vi "4CHDAQ - Check Text File Name.vi"(11 "path":path) -> (3 "Error Type":i32)   [LabVIEW 2015]
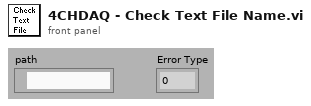
[diagram p1: front panel]
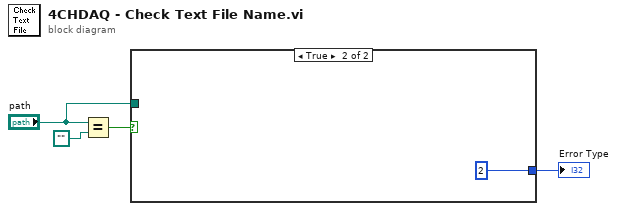
[diagram p0: block diagram]
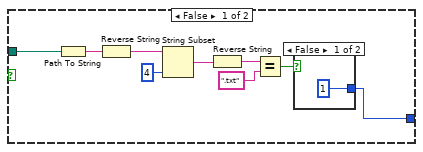
[diagram p2: hidden frame]
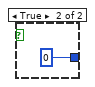
[diagram p3: hidden frame]
diagram:
  n1 = Equal?(x="path", y=path "") -> (x = y?=w3:bool)
  n2 = case shown="True" w3 {
    tunnel: [w5 2] -> w1
    tunnel: "path" -> [w6 _]
    frame False {
      n3 = Path To String(path=w6) -> (string=w13:string)
      n4 = Reverse String(1:w13) -> (0:w12:string)
      n5 = String Subset(string=w12, length (rest)=4 ("length (rest)")) -> (substring=w10:string)  [unwired: 1 in]
      n6 = Reverse String(1:w10) -> (0:w9:string)
      n7 = Equal?(x=w9, y=".txt") -> (x = y?=w7:bool)
      n8 = case shown="False" w7 {
        tunnel: [1 0] -> w5
        frame False {
        }
        frame True {
        }
      }
    }
    frame True {
    }
  }
  "Error Type" <- w1
